vi "SW_Generate_Color_Ramp.vi"(1 "Colors rel. pos.":dbl[](array[numeric]), 2 "Colors array":u32[](array[colorbox])=[16711680, 16773418, 6618880, 9567230, 255]) -> (0 "Colors array":u32[](array[colorbox]))   [LabVIEW 2016]
panel:
  out "Color array size":i32
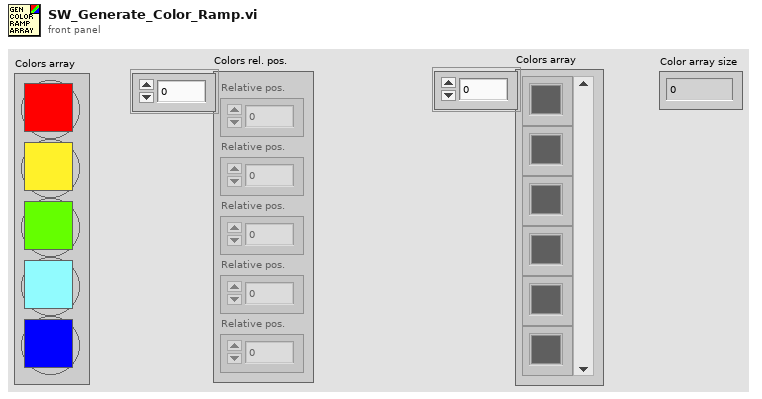
[diagram p1: front panel]
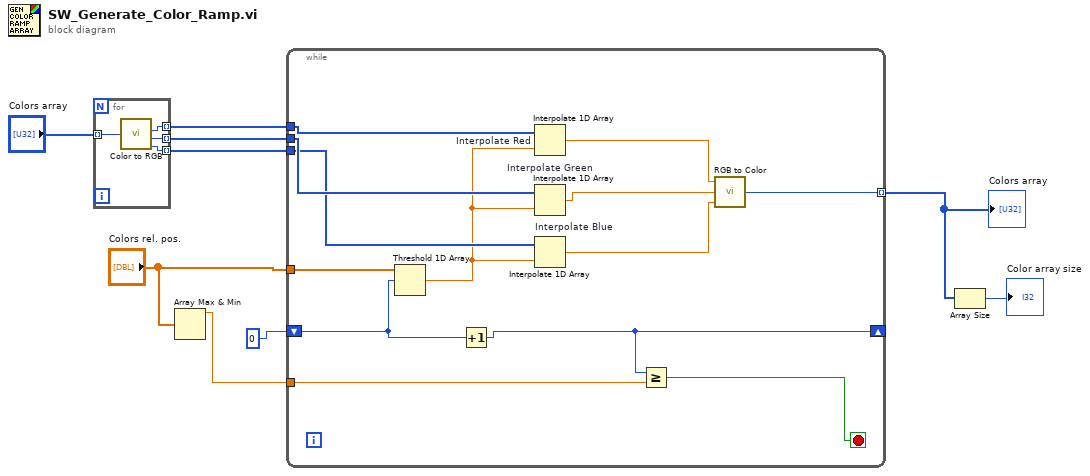
[diagram p0: block diagram]
diagram:
  n1 = for {
    tunnel: [w13] -> w8 mode=indexing
    tunnel: [w12] -> w7 mode=indexing
    tunnel: [w11] -> w6 mode=indexing
    tunnel: "Colors array" -> [w10] mode=indexing
    n2 = call <vilib>:"Color to RGB.vi"("Color"=w10) -> ("R"=w13:u8, "G"=w12:u8, "B"=w11:u8)  [unwired: 1 out]
  }
  n3 = Array Max & Min(array="Colors rel. pos.") -> (max value=w1:dbl)  [unwired: 3 out]
  n4 = while {
    tunnel: "Colors rel. pos." -> [w26]
    tunnel: w8 -> [w25]
    tunnel: w7 -> [w24]
    tunnel: w6 -> [w23]
    tunnel: [w18] -> w4 mode=indexing
    shift-right: [w16] -> _
    shift-left: 0 -> [w17]
    tunnel: w1 -> [w14]
    stop <- w15 stop-if-true
    n5 = Threshold 1D Array(2:w17, 3:w26) -> (0:w22:dbl)  [unwired: 1 in]
    n6 = Increment(x=w17) -> (x+1=w16:i32)
    n7 = Interpolate 1D Array "Interpolate Red"(1:w22, 2:w25) -> (0:w21:dbl)
    n8 = Interpolate 1D Array "Interpolate Green"(1:w22, 2:w24) -> (0:w20:dbl)
    n9 = Interpolate 1D Array "Interpolate Blue"(1:w22, 2:w23) -> (0:w19:dbl)
    n10 = Greater Or Equal?(x=w16, y=w14) -> (x >= y?=w15:bool)
    n11 = call <vilib>:"RGB to Color.vi"("B"=w19, "G"=w20, "R"=w21) -> ("Color"=w18:u32)
  }
  "Colors array" <- w4
  n12 = Array Size(array=w4) -> (size(s)=→"Color array size":i32)
